vi "Manual Build SM.vi"(8 "error in":errorcluster, 11 "Path to VIPB File":path=path "C:/Users/patrick/Documents/GitHub/PPMS-Monitor-and-Control/build support/PPMS Instrument.vipb") -> (0 "error out":errorcluster)   [LabVIEW 2019]
doc: "JKI State Machine version of Manual Build.vi that also builds a VIPM *.vip file.\n\nUse to build a (0) VI Package, (1) Application (EXE), (2) Installer, and finally (3) a single 7z self-extracting installer file.\n\n<b>Path to VIPB File</b> points to the VI Package Build spec you would like to build. Searchs for *.lvproj."
uses:
  <vilib>/AppBuilder/AB_API_Simple/NI_App_Builder_API.lvlib
  <vilib>/JKI/VIPM API/VIPM API_vipm_api.lvlib
  <userlib>/LevyLab/Progress Bar/ProgressBar/ProgressBar.lvclass
  <vilib>/AppBuilder/AB_API_Simple/Build (path).vi
  <vilib>/AppBuilder/AB_API_Simple/Set Build Specification Version (path).vi
  PostBuildSupport/PostBuildSupport.lvclass
  ProjectItem/ProjectItem.lvclass
  Build/Build.lvlib
panel:
  out "Current State":string="Exit"
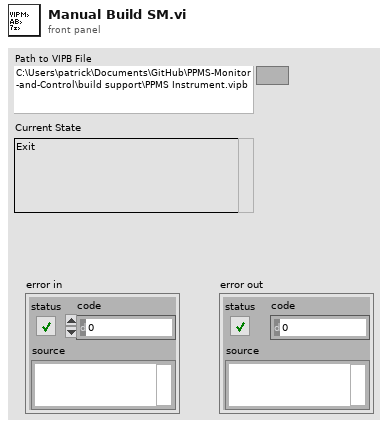
[diagram p1: front panel]
types:
  T1 = enum32{"Invalid", "Standard", "Closed", "Hidden", "Minimized", "Maximized"}
  T2 = enum32{"invalid app kind", "Development System", "Run Time System", "Student Edition", "Embedded LabVIEW", "Evaluation", "Custom"}
  T3 = cluster{"Core":cluster{"Current VI Reference":refnum<vi>, "Close Panel on Exit?":bool}, "ProgressBar":refnum<class "ProgressBar.lvclass">, "Product Name":string, "Package Version":string, "Package Source Folder":path, "Path to Project":path, "Path to VIPB File":path, "Output Package File Path":path}
  T4 = cluster{"Current VI Reference":refnum<vi>, "Close Panel on Exit?":bool}
  T5 = typedef "VIPM API_vipm_api.lvlib/VI Package Build Spec Data Cluster_vipm_api.ctl" = cluster{"Package Version":T6, "Product Name":string, "Company Name":string, "Author Name (Person or Company)":string, "Product Homepage (URL)":string, "Legal Copyright":string, "License Agreement Name":string, "Product Description Summary":string, "Product Description":string, "Release Notes - Change Log":string}
  T6 = typedef "VIPM API_vipm_api.lvlib/Version Info Cluster_vipm_api.ctl" = cluster{"major":u32, "minor":u32, "patch":u32, "build":u32}
  T7 = typedef "Build.lvlib/Build Spec--cluster.ctl" = cluster{"Name":string, "Type":string, "Version":string}
  T8 = typedef "NI_App_Builder_API.lvlib/Build Specification Version.ctl" = cluster{"Major":u16, "Minor":u16, "Fix":u16, "Build":u16}
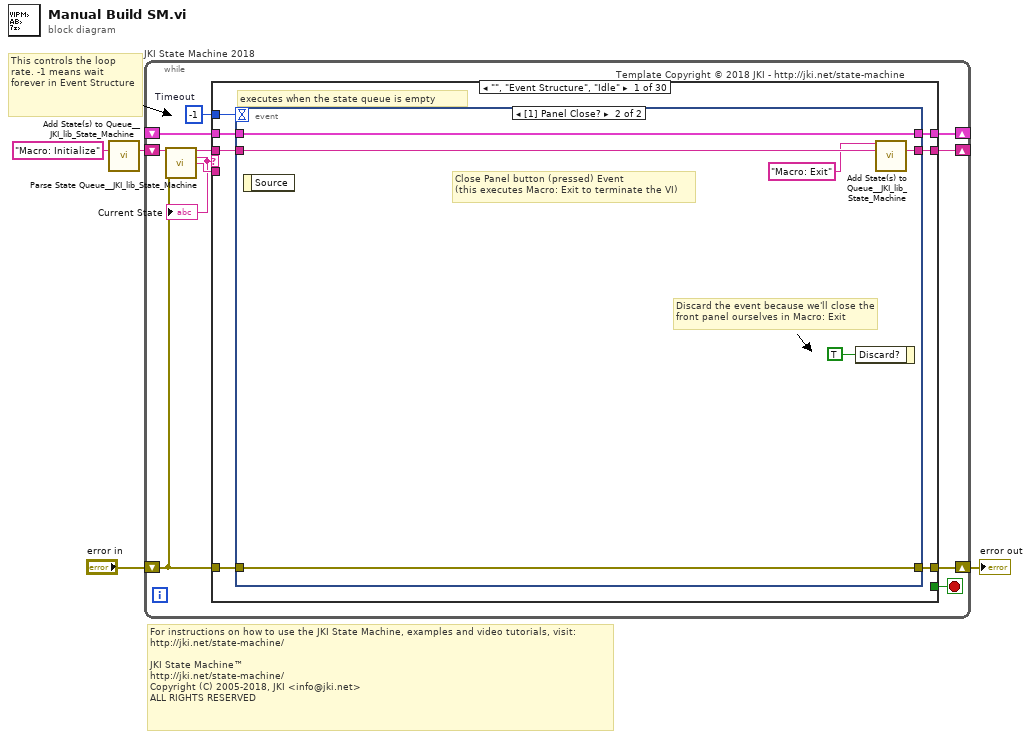
[diagram p0: block diagram]
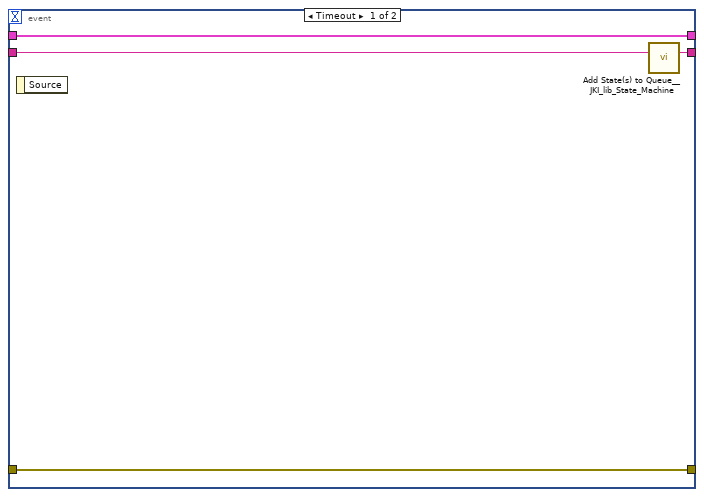
[diagram p2: hidden frame]
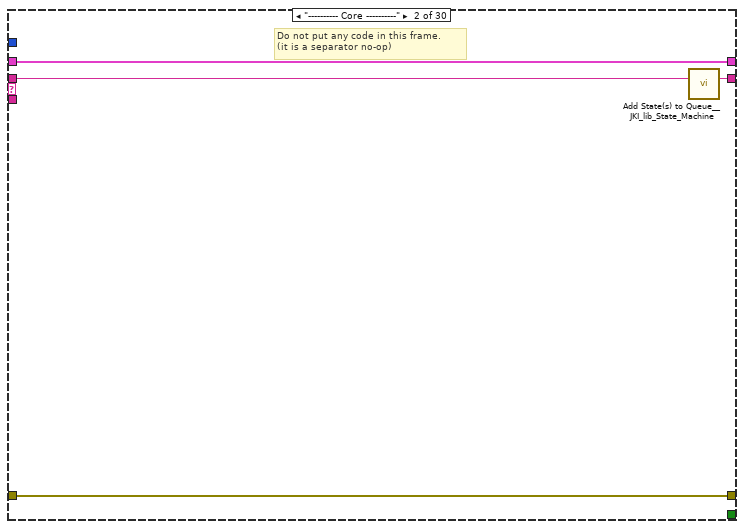
[diagram p3: hidden frame]
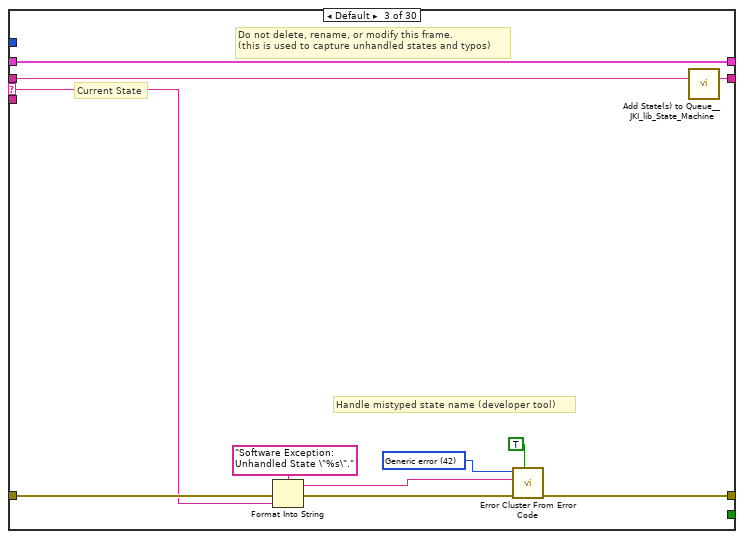
[diagram p4: hidden frame]
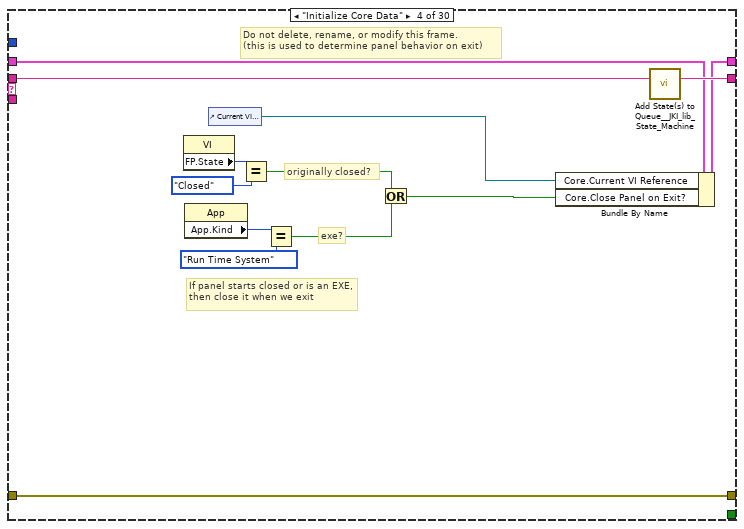
[diagram p5: hidden frame]
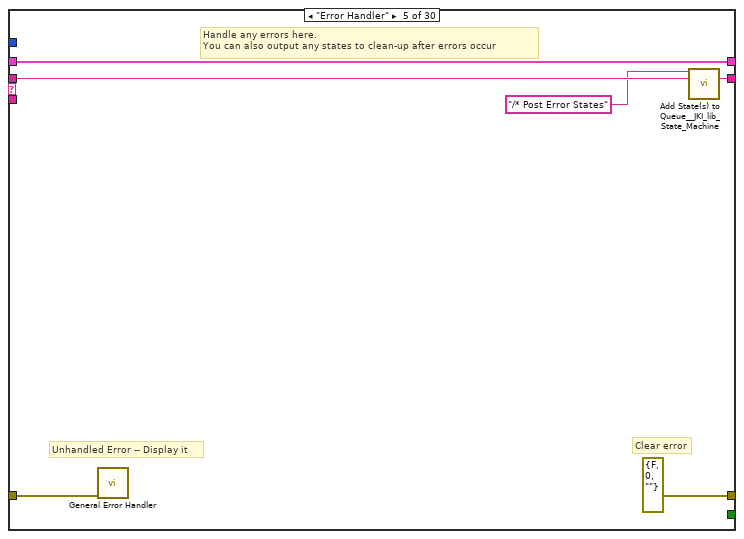
[diagram p6: hidden frame]
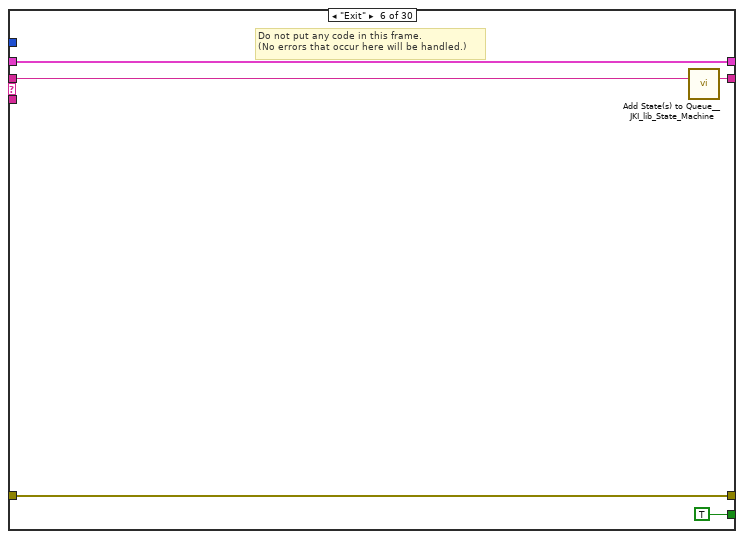
[diagram p7: hidden frame]
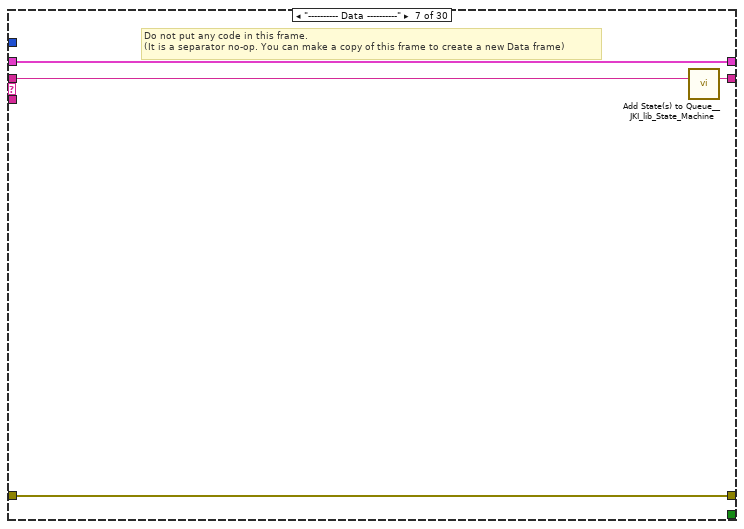
[diagram p8: hidden frame]
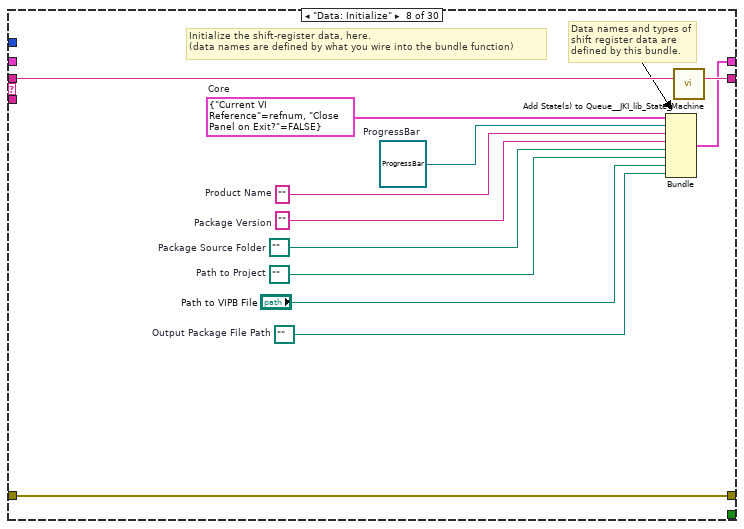
[diagram p9: hidden frame]
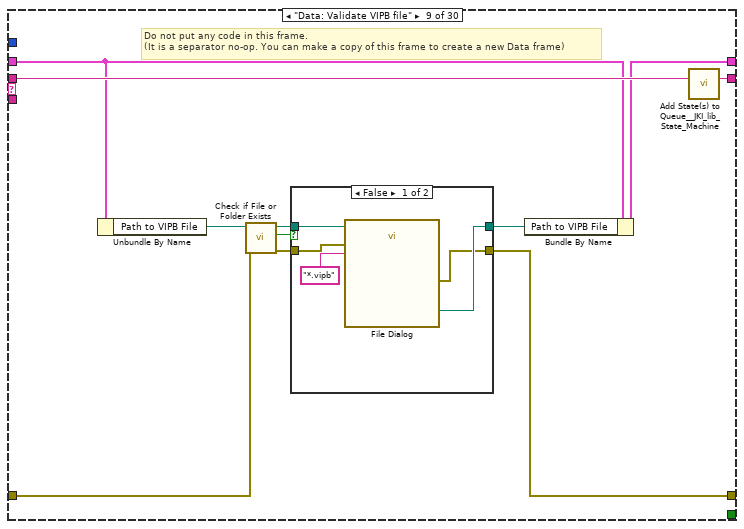
[diagram p10: hidden frame]
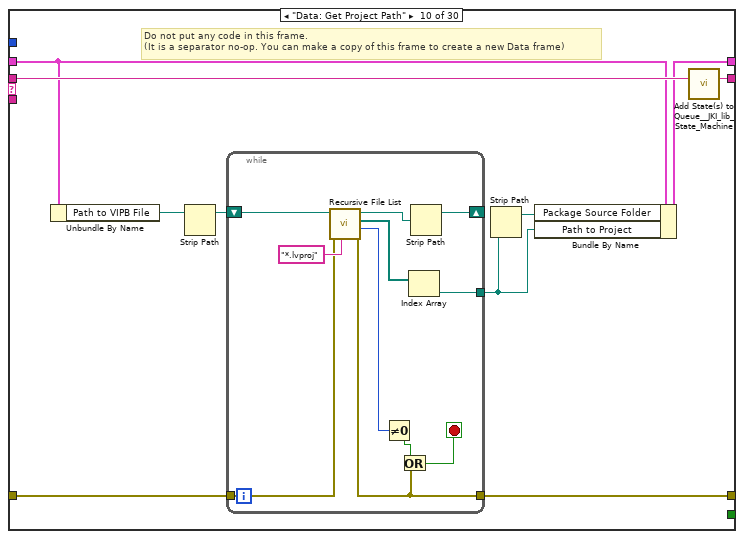
[diagram p12: hidden frame]
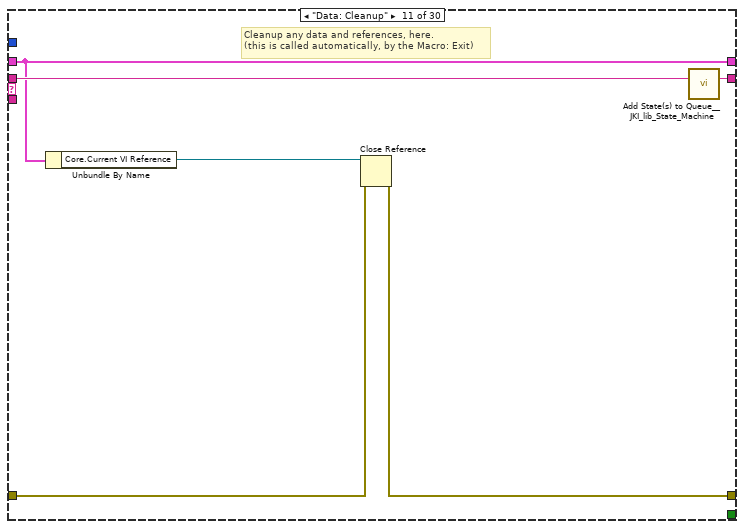
[diagram p13: hidden frame]
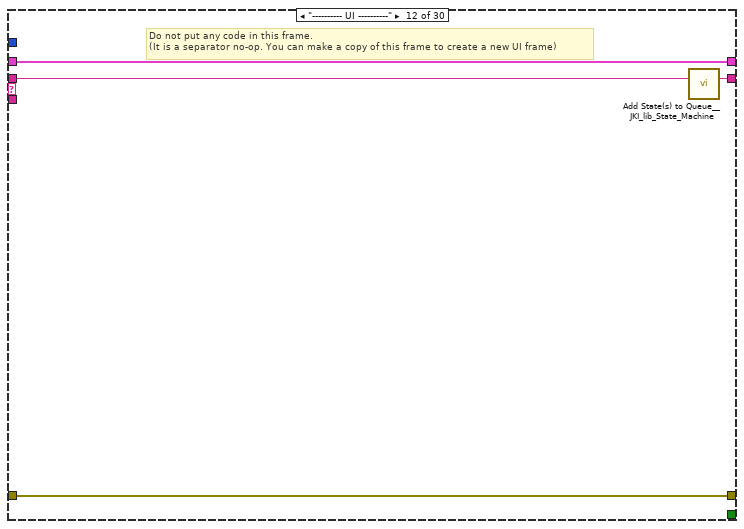
[diagram p14: hidden frame]
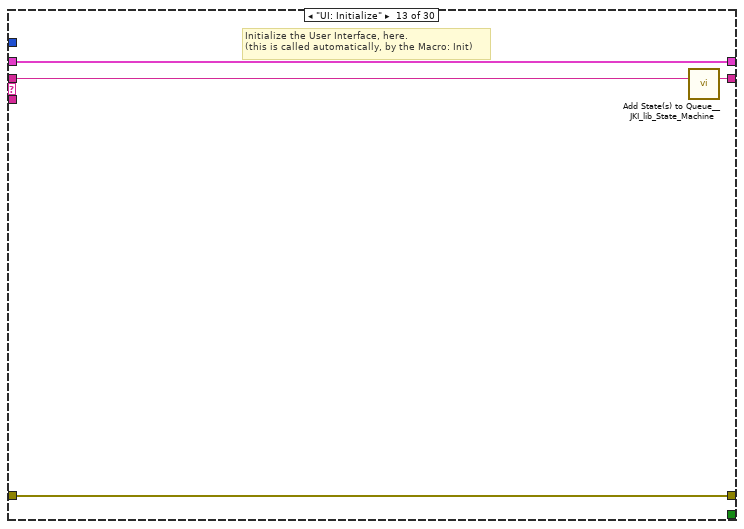
[diagram p15: hidden frame]
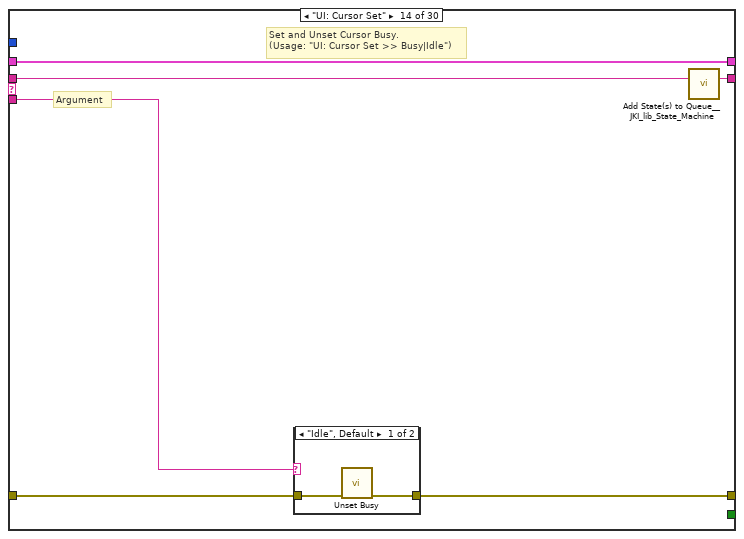
[diagram p16: hidden frame]
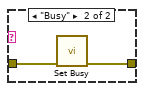
[diagram p17: hidden frame]
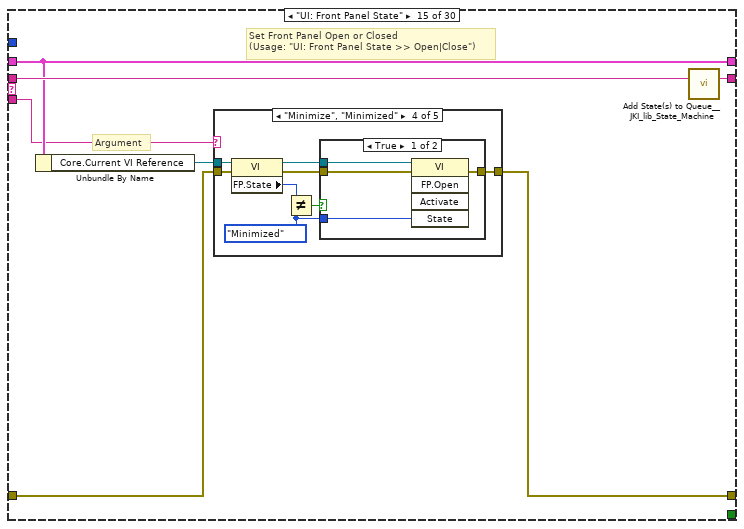
[diagram p18: hidden frame]
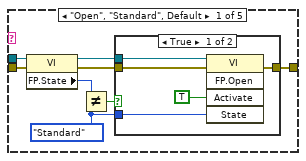
[diagram p19: hidden frame]
diagram:
  # "For instructions on how to use the JKI State Machine, examples and video tutorials, visit:\nhttp://jki.net/state-machine/\n\nJKI State Machine™\nhttp://jki.net/state-machine/\nCopyright (C) 2005-2018, JKI <info@jki.net>\nALL RIGHTS RESERVED"
  # "This controls the loop rate. -1 means wait forever in Event Structure"
  n1 = call <vilib>:"Add State(s) to Queue__JKI_lib_State_Machine.vi"("State(s) in (\"\")"="Macro: Initialize") -> ("States Out"=w4:string)  [unwired: 14 in]
  n2 = while "JKI State Machine 2018" {
    shift-right: [w9] -> _
    shift-left: _ -> [w8]
    shift-right: [w12] -> w2
    shift-left: "error in" -> [w6]
    shift-right: [w11] -> _
    shift-left: w4 -> [w13]
    stop <- w10 stop-if-true
    w7 = -1  # Timeout
    # "Template Copyright © 2018 JKI - http://jki.net/state-machine"
    n3 = call <vilib>:"Parse State Queue__JKI_lib_State_Machine.vi"("State Queue"=w13, "Error In (no error)"=w6) -> ("Remaining States"=w15:string, "Current State"=w5:string, "Arguments"=w14:string)  [unwired: 11 in]
    "Current State" <- w5
    n4 = case shown="\"\", \"Event Structure\", \"Idle\"" w5 {
      selector: w5 -> [_ _ w37 _ _ _ _ _ _ _ _ _ _ _ _ _ _ _ _ _ _ _ _ _ _ _ _ _ w326 _]
      tunnel: w15 -> [w22 w36 w41 w60 w66 w71 w75 w87 w98 w115 w132 w136 w140 w146 w157 w226 w231 w236 w247 w251 w266 w274 w278 w286 w294 w303 w307 w319 w331 w339]
      tunnel: w14 -> [_ _ _ _ _ _ _ _ _ _ _ _ _ w141 w151 _ _ _ _ _ _ _ _ _ _ w295 _ w311 w321 _]
      tunnel: w8 -> [w20 w33 w39 w53 w63 w69 w72 _ w91 w112 w127 w133 w138 w144 w153 w223 w228 w233 w244 w249 w256 w267 w276 w279 w291 w300 w305 w317 w329 w337]
      tunnel: [w19 w34 w43 w57 errorcluster {"status"=FALSE, "code"=0, "source"=""} ("error out") w68 w73 w84 w90 w111 w128 w134 w137 w142 w154 w224 w229 w234 w245 w248 w253 w271 w275 w282 w287 w297 w304 w316 w328 w333] -> w12
      tunnel: w6 -> [w18 w34 w42 w57 w62 w68 w73 w84 w88 w110 w129 w134 w137 w143 w155 w224 w229 w234 w245 w248 w252 w270 w275 w281 w288 w296 w304 w312 w327 _]
      tunnel: [w21 w35 w40 w59 w65 w70 w74 w86 w97 w114 w131 w135 w139 w145 w156 w225 w230 w235 w246 w250 w265 w273 w277 w285 w293 w302 w306 w318 w330 w338] -> w11
      tunnel: [_ _ _ _ _ TRUE _ _ _ _ _ _ _ _ _ _ _ _ _ _ _ _ _ _ _ _ _ _ _ _] -> w10
      tunnel: [w17 w33 w39 w58 w63 w69 w72 w85 w92 w113 w127 w133 w138 w144 w153 w223 w228 w233 w244 w249 w257 w268 w276 w280 w292 w301 w305 w317 w329 w337] -> w9
      tunnel: w7 -> [w16 _ _ _ _ _ _ _ _ _ _ _ _ _ _ _ _ _ _ _ _ _ _ _ _ _ _ _ _ _]
      frame "", "Event Structure", "Idle" {
        # "executes when the state queue is empty"
        n5 = event shown="[1] Panel Close?" {
          selector: _ -> [_ _]
          dyn-events: _ -> [_ _]
          timeout: w16 -> [_ _]
          tunnel: w22 -> [w26 w32]
          tunnel: [w25 w31] -> w21
          tunnel: w20 -> [w23 w29]
          tunnel: [w24 w30] -> w19
          tunnel: w18 -> [w24 w30]
          tunnel: [w23 w29] -> w17
          event Timeout {
            n6 = event-data() -> ()  [unwired: 1 in, 1 out]
            n7 = call <vilib>:"Add State(s) to Queue__JKI_lib_State_Machine.vi"("State(s) in (\"\")"=w26) -> ("States Out"=w25:string)  [unwired: 14 in]
          }
          event Panel Close? {
            # "Discard the event because we'll close the front panel ourselves in Macro: Exit"
            # "Close Panel button (pressed) Event\n(this executes Macro: Exit to terminate the VI)"
            n8 = event-data() -> ()  [unwired: 1 in, 1 out]
            n9 = event-data("Discard?"=TRUE) -> ()  [unwired: 1 in, 1 out]
            n10 = call <vilib>:"Add State(s) to Queue__JKI_lib_State_Machine.vi"("State(s) in Front (\"\")"="Macro: Exit", "State(s) in (\"\")"=w32) -> ("States Out"=w31:string)  [unwired: 13 in]
          }
        }
      }
      frame "---------- Core ----------" {
        # "Do not put any code in this frame.\n(it is a separator no-op)"
        n11 = call <vilib>:"Add State(s) to Queue__JKI_lib_State_Machine.vi"("State(s) in (\"\")"=w36) -> ("States Out"=w35:string)  [unwired: 14 in]
      }
      frame Default {
        w46 = 42 items=["No error", "Argument error", "Memory is full", "Out of zone", "End of file", "File already open", "Generic file I/O error", "File not found", "File permission error", "Disk is full", "Duplicate path", "Too many files open", "System feature not enabled", "Resource file not found", "Cannot add resource", "Resource not found", "Image not found", "Image memory error", "Pen does not exist", "Config type invalid", "Config token not found", "Config parse error", "Config memory error", "Bad external code format", "Bad external code offset", "External code not present", "Null window", "Destroy window error", "Null menu", "Print aborted", "Bad print record", "Print driver error", "Windows error during printing", "Memory error during printing", "Print dialog error", "Generic print error", "Invalid device refnum", "Device not found", "Device parameter error", "Device unit error", "Cannot open device", "Device call aborted", "Generic error", "Cancelled by user", "Object ID too low", "Object ID too high", "Object not in heap", "Unknown heap", "Unknown object (invalid DefProc)", "Unknown object (DefProc not in table)", "Message out of range", "Invalid (null) method", "Unknown message", "Manager call not supported", "Bad address", "Network operation in progress", "Network operation timed out", "Connection is busy", "Network attribute not supported", "Network error", "Address in use", "System out of memory", "Connection aborted", "Connection refused", "Not connected", "Already connected", "Connection closed", "Initialization error (interapplication manager)", "Bad occurrence", "Wait on unbound occurrence handler", "Occurrence queue overflow", "Datalog type conflict", "Unused", "Unrecognized type (interapplication manager)", "Memory corrupt", "Failed to make temporary DLL", "Old CIN version", "Drag socket not found", "Failed to load drop-object", "Failed to register OLE object", "Failed to release OLE object", "Format specifier type mismatch", "Unknown format specifier", "Too few format specifiers", "Too many format specifiers", "Scan failed", "Newer CIN version", "Error converting to variant", "Runtime menu error", "Password tampered", "Variant attribute not found", "Incompatible variant data type", "Event data is not available", "Event Store is not present", "Occurrence is not found", "Event Queue is not created", "Event info is not available", "Refnum passed is NULL", "Error retrieving Class GUID", "Error retrieving CoClass GUID", "Error retrieving TypeLib GUID.", "Bad built application magic bytes.", "Specific driver is different from the specific driver associated with the Logical Name.", "There is no session opened to the class driver.", "Max Error", "MAX - Error with config objects", "MAX - Error loading configuration", "MAX - Group not supported"]
        # "Current State"
        # "Do not delete, rename, or modify this frame.\n(this is used to capture unhandled states and typos)"
        # "Handle mistyped state name (developer tool)"
        n12 = Format Into String(format string="Software Exception: Unhandled State \"%s\"." ("message"), error in=w42, w37) -> (resulting string=w45:string, error out=w44:errorcluster)  [unwired: 1 in]
        n13 = call <vilib>:"Error Cluster From Error Code.vi"("show call chain? (False)"=TRUE, "error in (no error)"=w44, "error message (\"\")"=w45, "error code (0)"=w46) -> ("error out"=w43:errorcluster)  [unwired: 5 in]
        n14 = call <vilib>:"Add State(s) to Queue__JKI_lib_State_Machine.vi"("State(s) in (\"\")"=w41) -> ("States Out"=w40:string)  [unwired: 14 in]
      }
      frame "Initialize Core Data" {
        # "Do not delete, rename, or modify this frame.\n(this is used to determine panel behavior on exit)"
        # "originally closed?"
        # "exe?"
        # "If panel starts closed or is an EXE, then close it when we exit"
        n15 = property class="VI"() -> ("FP.State"=w50:T1)  [unwired: 2 in, 2 out]
        n16 = property class="App"() -> ("App.Kind"=w56:T2)  [unwired: 2 in, 2 out]
        n17 = control-ref of="Current VI Reference"() -> (w51:refnum<vi>)
        n18 = Equal?(x=w50, y=T1."Closed" ("Front Panel Window:State")) -> (x = y?=w48:bool)
        n19 = Equal?(x=w56, y=T2."Run Time System" ("Application:Kind")) -> (x = y?=w54:bool)
        n20 = Or(x=w48, y=w54) -> (x .or. y?=w52:bool)
        n21 = Bundle By Name(cluster=w53, "Core.Current VI Reference"=w51, "Core.Close Panel on Exit?"=w52) -> (w58:T3)
        n22 = call <vilib>:"Add State(s) to Queue__JKI_lib_State_Machine.vi"("State(s) in (\"\")"=w60) -> ("States Out"=w59:string)  [unwired: 14 in]
      }
      frame "Error Handler" {
        # "Unhandled Error -- Display it"
        # "Handle any errors here.\nYou can also output any states to clean-up after errors occur"
        # "Clear error"
        n23 = call <vilib>:"General Error Handler.vi"("error in (no error)"=w62) -> ()  [unwired: 10 in, 5 out]
        n24 = call <vilib>:"Add State(s) to Queue__JKI_lib_State_Machine.vi"("State(s) in Front (\"\")"="/* Post Error States", "State(s) in (\"\")"=w66) -> ("States Out"=w65:string)  [unwired: 13 in]
      }
      frame "Exit" {
        # "Do not put any code in this frame.\n(No errors that occur here will be handled.)"
        n25 = call <vilib>:"Add State(s) to Queue__JKI_lib_State_Machine.vi"("State(s) in (\"\")"=w71) -> ("States Out"=w70:string)  [unwired: 14 in]
      }
      frame "---------- Data ----------" {
        # "Do not put any code in this frame.\n(It is a separator no-op. You can make a copy of this frame to create a new Data frame)"
        n26 = call <vilib>:"Add State(s) to Queue__JKI_lib_State_Machine.vi"("State(s) in (\"\")"=w75) -> ("States Out"=w74:string)  [unwired: 14 in]
      }
      frame "Data: Initialize" {
        w77 = path ""  # Path to Project
        w78 = refnum<class "ProgressBar.lvclass"> refnum  # ProgressBar
        w79 = path ""  # Output Package File Path
        w81 = ""  # Package Version
        w82 = ""  # Product Name
        w80 = path ""  # Package Source Folder
        w83 = T4 {"Current VI Reference"=refnum, "Close Panel on Exit?"=FALSE}  # Core
        # "Data names and types of shift register data are defined by this bundle."
        # "Initialize the shift-register data, here.\n(data names are defined by what you wire into the bundle function)"
        n27 = Bundle("Core"=w83, "ProgressBar"=w78, "Product Name"=w82, "Package Version"=w81, "Package Source Folder"=w80, "Path to Project"=w77, "Path to VIPB File"="Path to VIPB File", "Output Package File Path"=w79) -> (w85:T3)  [unwired: 1 in]
        n28 = call <vilib>:"Add State(s) to Queue__JKI_lib_State_Machine.vi"("State(s) in (\"\")"=w87) -> ("States Out"=w86:string)  [unwired: 14 in]
      }
      frame "Data: Validate VIPB file" {
        # "Do not put any code in this frame.\n(It is a separator no-op. You can make a copy of this frame to create a new Data frame)"
        n29 = Unbundle By Name(w91) -> ("Path to VIPB File"=w95:path)
        n30 = call <vilib>:"Check if File or Folder Exists.vi"("error in (no error)"=w88, "path"=w95) -> ("error out"=w89:errorcluster, "file or folder exists?"=w96:bool, "dup path"=w94:path)  [unwired: 7 in]
        n31 = case shown="False" w96 {
          tunnel: w94 -> [w103 w105]
          tunnel: [w102 w105] -> w93
          tunnel: [w99 w104] -> w90
          tunnel: w89 -> [w101 w104]
          frame False {
            n32 = call "File Dialog"("start path"=w103, "error in"=w101, "pattern (all files)"="*.vipb") -> ("selected path"=w102:path, "error out"=w99:errorcluster)  [unwired: 9 in, 2 out]
          }
          frame True {
          }
        }
        n33 = Bundle By Name(cluster=w91, "Path to VIPB File"=w93) -> (w92:T3)
        n34 = call <vilib>:"Add State(s) to Queue__JKI_lib_State_Machine.vi"("State(s) in (\"\")"=w98) -> ("States Out"=w97:string)  [unwired: 14 in]
      }
      frame "Data: Get Project Path" {
        # "Do not put any code in this frame.\n(It is a separator no-op. You can make a copy of this frame to create a new Data frame)"
        n35 = Unbundle By Name(w112) -> ("Path to VIPB File"=w109:path)
        n36 = Strip Path(path=w109) -> (stripped path=w108:path)  [unwired: 1 out]
        n37 = while {
          tunnel: [w119] -> w111
          tunnel: w110 -> [w121]
          shift-right: [w124] -> _
          shift-left: w108 -> [w120]
          tunnel: [w122] -> w107
          stop <- w117 stop-if-true
          n38 = call <vilib>:"Recursive File List.vi"("pattern"="*.lvproj", "error in (no error)"=w121, "Folder Path"=w120) -> ("error out"=w119:errorcluster, "Number of Files"=w125:i32, "All Files in Dir"=w116:path[], "dup Folder Path"=w123:path)  [unwired: 4 in, 1 out]
          n39 = Not Equal To 0?(x=w125) -> (x != 0?=w118:bool)
          n40 = Or(x=w118, y=w119) -> (x .or. y?=w117:bool)
          n41 = Index Array(array=w116) -> (element=w122:path)  [unwired: 1 in]
          n42 = Strip Path(path=w123) -> (stripped path=w124:path)  [unwired: 1 out]
        }
        n43 = Strip Path(path=w107) -> (stripped path=w106:path)  [unwired: 1 out]
        n44 = Bundle By Name(cluster=w112, "Package Source Folder"=w106, "Path to Project"=w107) -> (w113:T3)
        n45 = call <vilib>:"Add State(s) to Queue__JKI_lib_State_Machine.vi"("State(s) in (\"\")"=w115) -> ("States Out"=w114:string)  [unwired: 14 in]
      }
      frame "Data: Cleanup" {
        # "Cleanup any data and references, here.\n(this is called automatically, by the Macro: Exit)"
        n46 = Unbundle By Name(w127) -> ("Core.Current VI Reference"=w130:refnum<vi>)
        n47 = Close Reference(reference=w130, error in (no error)=w129) -> (error out=w128:errorcluster)
        n48 = call <vilib>:"Add State(s) to Queue__JKI_lib_State_Machine.vi"("State(s) in (\"\")"=w132) -> ("States Out"=w131:string)  [unwired: 14 in]
      }
      frame "---------- UI ----------" {
        # "Do not put any code in this frame.\n(It is a separator no-op. You can make a copy of this frame to create a new UI frame)"
        n49 = call <vilib>:"Add State(s) to Queue__JKI_lib_State_Machine.vi"("State(s) in (\"\")"=w136) -> ("States Out"=w135:string)  [unwired: 14 in]
      }
      frame "UI: Initialize" {
        # "Initialize the User Interface, here.\n(this is called automatically, by the Macro: Init)"
        n50 = call <vilib>:"Add State(s) to Queue__JKI_lib_State_Machine.vi"("State(s) in (\"\")"=w140) -> ("States Out"=w139:string)  [unwired: 14 in]
      }
      frame "UI: Cursor Set" {
        # "Argument"
        # "Set and Unset Cursor Busy.\n(Usage: \"UI: Cursor Set >> Busy|Idle\")"
        n51 = case shown="\"Idle\", Default" w141 {
          tunnel: w143 -> [w148 w150]
          tunnel: [w147 w149] -> w142
          frame "Idle", Default {
            n52 = call <vilib>:"Unset Busy.vi"("error in (no error)"=w148) -> ("error out"=w147:errorcluster)  [unwired: 10 in]
          }
          frame "Busy" {
            n53 = call <vilib>:"Set Busy.vi"("error in (no error)"=w150) -> ("error out"=w149:errorcluster)  [unwired: 9 in, 1 out]
          }
        }
        n54 = call <vilib>:"Add State(s) to Queue__JKI_lib_State_Machine.vi"("State(s) in (\"\")"=w146) -> ("States Out"=w145:string)  [unwired: 14 in]
      }
      frame "UI: Front Panel State" {
        # "Argument"
        # "Set Front Panel Open or Closed\n(Usage: \"UI: Front Panel State >> Open|Close\")"
        n55 = Unbundle By Name(w153) -> ("Core.Current VI Reference"=w152:refnum<vi>)
        n56 = case shown="\"Minimize\", \"Minimized\"" w151 {
          tunnel: w155 -> [w163 w178 w189 w202 w215]
          tunnel: [w165 w179 w191 w204 w217] -> w154
          tunnel: w152 -> [w164 w176 w190 w203 w216]
          frame "Open", "Standard", Default {
            w158 = T1."Standard" ("State")
            n57 = property class="VI"(reference=w164, error in=w163) -> (reference out=w161:refnum<vi>, error out=w162:errorcluster, "FP.State"=w160:T1)
            n58 = Not Equal?(x=w160, y=w158) -> (x != y?=w159:bool)
            n59 = case shown="True" w159 {
              tunnel: [w169 w171] -> w165
              tunnel: w162 -> [w168 w171]
              tunnel: w161 -> [w167 _]
              tunnel: w158 -> [w166 _]
              frame True {
                n60 = invoke class="VI" method="FP.Open"(reference=w167, error in=w168, "Activate"=TRUE, "State"=w166) -> (error out=w169:errorcluster)  [unwired: 1 in, 4 out]
              }
              frame False {
              }
            }
          }
          frame "Close", "Closed" {
            n61 = property class="VI"(reference=w176, error in=w178) -> (reference out=w175:refnum<vi>, error out=w177:errorcluster, "FP.State"=w173:T1)
            n62 = Not Equal?(x=w173, y=T1."Closed" ("Front Panel Window:State")) -> (x != y?=w172:bool)
            n63 = case shown="True" w172 {
              tunnel: [w180 w183] -> w179
              tunnel: w177 -> [w180 w182]
              tunnel: w175 -> [_ w181]
              frame False {
              }
              frame True {
                n64 = invoke class="VI" method="FP.Close"(reference=w181, error in=w182) -> (error out=w183:errorcluster)  [unwired: 1 in, 2 out]
              }
            }
          }
          frame "Hidden", "Hide" {
            w184 = T1."Hidden" ("State")
            n65 = property class="VI"(reference=w190, error in=w189) -> (reference out=w187:refnum<vi>, error out=w188:errorcluster, "FP.State"=w186:T1)
            n66 = Not Equal?(x=w186, y=w184) -> (x != y?=w185:bool)
            n67 = case shown="True" w185 {
              tunnel: [w195 w196] -> w191
              tunnel: w188 -> [w194 w196]
              tunnel: w187 -> [w193 _]
              tunnel: w184 -> [w192 _]
              frame True {
                n68 = invoke class="VI" method="FP.Open"(reference=w193, error in=w194, "State"=w192) -> (error out=w195:errorcluster)  [unwired: 2 in, 4 out]
              }
              frame False {
              }
            }
          }
          frame "Minimize", "Minimized" {
            w197 = T1."Minimized" ("State")
            n69 = property class="VI"(reference=w203, error in=w202) -> (reference out=w200:refnum<vi>, error out=w201:errorcluster, "FP.State"=w199:T1)
            n70 = Not Equal?(x=w199, y=w197) -> (x != y?=w198:bool)
            n71 = case shown="True" w198 {
              tunnel: [w208 w209] -> w204
              tunnel: w201 -> [w207 w209]
              tunnel: w200 -> [w206 _]
              tunnel: w197 -> [w205 _]
              frame True {
                n72 = invoke class="VI" method="FP.Open"(reference=w206, error in=w207, "State"=w205) -> (error out=w208:errorcluster)  [unwired: 2 in, 4 out]
              }
              frame False {
              }
            }
          }
          frame "Maximize", "Maximized" {
            w210 = T1."Maximized" ("State")
            n73 = property class="VI"(reference=w216, error in=w215) -> (reference out=w213:refnum<vi>, error out=w214:errorcluster, "FP.State"=w212:T1)
            n74 = Not Equal?(x=w212, y=w210) -> (x != y?=w211:bool)
            n75 = case shown="True" w211 {
              tunnel: [w221 w222] -> w217
              tunnel: w214 -> [w220 w222]
              tunnel: w213 -> [w219 _]
              tunnel: w210 -> [w218 _]
              frame True {
                n76 = invoke class="VI" method="FP.Open"(reference=w219, error in=w220, "State"=w218) -> (error out=w221:errorcluster)  [unwired: 2 in, 4 out]
              }
              frame False {
              }
            }
          }
        }
        n77 = call <vilib>:"Add State(s) to Queue__JKI_lib_State_Machine.vi"("State(s) in (\"\")"=w157) -> ("States Out"=w156:string)  [unwired: 14 in]
      }
      frame "---------- Macro ----------" {
        # "Do not put any code in this frame.\n(It is a separator no-op. You can make a copy of this frame to create a new Macro frame)"
        n78 = call <vilib>:"Add State(s) to Queue__JKI_lib_State_Machine.vi"("State(s) in (\"\")"=w226) -> ("States Out"=w225:string)  [unwired: 14 in]
      }
      frame "Macro: Initialize" {
        w227 = "Data: Initialize\nInitialize Core Data\nUI: Initialize\nUI: Front Panel State >> Open\nData: Validate VIPB file\n\nMacro: Build\nMacro: Exit"  # Data: Initialize Initialize Core Data UI: Initialize UI: Front Panel State >> Open Data: Validate VIPB file  Macro: Build Macro: Exit
        # "Initialization Macro\n(This is called once, when the VI starts)"
        n79 = call <vilib>:"Add State(s) to Queue__JKI_lib_State_Machine.vi"("State(s) in Front (\"\")"=w227, "State(s) in (\"\")"=w231) -> ("States Out"=w230:string)  [unwired: 13 in]
      }
      frame "Macro: Build" {
        # "Initialization Macro\n(This is called once, when the VI starts)"
        n80 = call <vilib>:"Add State(s) to Queue__JKI_lib_State_Machine.vi"("State(s) in Front (\"\")"="Data: Get Project Path\nVIPM: Read VIPB\nVIPM: Build\nAB: Update Version >> Application\nAB: Update Version >> Installer\nAB: Build >> Application\nAB: Build >> Installer\nAB: Build exe", "State(s) in (\"\")"=w236) -> ("States Out"=w235:string)  [unwired: 13 in]
      }
      frame "Macro: Exit" {
        # "Exit Macro\n(This is called once, when the VI exits)"
        n81 = Unbundle By Name(w244) -> ("Core.Close Panel on Exit?"=w243:bool)
        n82 = Select(t="UI: Front Panel State >> Close", s=w243, f="") -> (s? t:f=w240:string)
        n83 = call <vilib>:"Add State(s) to Queue__JKI_lib_State_Machine.vi"("State(s) in Front (\"\")"="", "State(s) in (\"\")"=w240, "State(s) at Back (\"\")"="Data: Cleanup\nExit") -> ("States Out"=w238:string)  [unwired: 12 in]
        n84 = call <vilib>:"Add State(s) to Queue__JKI_lib_State_Machine.vi"("State(s) in Front (\"\")"=w238, "State(s) in (\"\")"=w247) -> ("States Out"=w246:string)  [unwired: 13 in]
      }
      frame "---------- VIPM ----------" {
        # "Template Separator\n(You can make a copy of, or modify, this frame)"
        n85 = call <vilib>:"Add State(s) to Queue__JKI_lib_State_Machine.vi"("State(s) in (\"\")"=w251) -> ("States Out"=w250:string)  [unwired: 14 in]
      }
      frame "VIPM: Read VIPB" {
        # "Your code here.\n(You can make a copy of, or modify, this frame)"
        n86 = Unbundle By Name(w256) -> ("Path to VIPB File"=w259:path)
        n87 = call <vilib>:"Read VI Package Build Spec_vipm_api.vi"("error in (no error)"=w252, "Path to VIPB File"=w259) -> ("error out"=w253:errorcluster, "VI Package Build Spec Data"=w264:T5)  [unwired: 8 in]
        n88 = Unbundle By Name(w264) -> ("Package Version.major"=w255:u32, "Package Version.minor"=w263:u32, "Package Version.patch"=w262:u32, "Package Version.build"=w261:u32, "Product Name"=w254:string)
        n89 = Format Into String(format string="%d.%d.%d.%d", w255, w263, w262, w261) -> (resulting string=w258:string)  [unwired: 2 in, 1 out]
        n90 = Bundle By Name(cluster=w256, "Package Version"=w258, "Product Name"=w254) -> (w257:T3)
        n91 = call <vilib>:"Add State(s) to Queue__JKI_lib_State_Machine.vi"("State(s) in (\"\")"=w266) -> ("States Out"=w265:string)  [unwired: 14 in]
      }
      frame "VIPM: Build" {
        # "Your code here.\n(You can make a copy of, or modify, this frame)"
        n92 = Unbundle By Name(w267) -> ("Path to VIPB File"=w272:path)
        n93 = call <vilib>:"Build VI Package_vipm_api.vi"("error in (no error)"=w270, "Path to VIPB File"=w272) -> ("error out"=w271:errorcluster, "Build Output"=w269:path)  [unwired: 8 in]
        n94 = Bundle By Name(cluster=w267, "Output Package File Path"=w269) -> (w268:T3)
        n95 = call <vilib>:"Add State(s) to Queue__JKI_lib_State_Machine.vi"("State(s) in (\"\")"=w274) -> ("States Out"=w273:string)  [unwired: 14 in]
      }
      frame "---------- ProgressBar ----------" {
        # "Template Separator\n(You can make a copy of, or modify, this frame)"
        n96 = call <vilib>:"Add State(s) to Queue__JKI_lib_State_Machine.vi"("State(s) in (\"\")"=w278) -> ("States Out"=w277:string)  [unwired: 14 in]
      }
      frame "ProgressBar: Initialize" {
        # "Do not put any code in this frame.\n(It is a separator no-op. You can make a copy of this frame to create a new Data frame)"
        n97 = Unbundle By Name(w279) -> ("ProgressBar"=w284:refnum<class "ProgressBar.lvclass">)
        n98 = call <userlib>:"Initialize ProgressBar.vi"("error in (no error)"=w281, "ProgressBar in"=w284) -> ("error out"=w282:errorcluster, "ProgressBar out"=w283:refnum<class "ProgressBar.lvclass">)  [unwired: 8 in]
        n99 = Bundle By Name(cluster=w279, "ProgressBar"=w283) -> (w280:T3)
        n100 = call <vilib>:"Add State(s) to Queue__JKI_lib_State_Machine.vi"("State(s) in (\"\")"=w286) -> ("States Out"=w285:string)  [unwired: 14 in]
      }
      frame "ProgressBar: Destroy" {
        # "Do not put any code in this frame.\n(It is a separator no-op. You can make a copy of this frame to create a new Data frame)"
        n101 = Unbundle By Name(w291) -> ("ProgressBar"=w290:refnum<class "ProgressBar.lvclass">)
        n102 = call <userlib>:"Destroy ProgressBar.vi"("error in (no error)"=w288, "ProgressBar in"=w290) -> ("error out"=w287:errorcluster, "ProgressBar out"=w289:refnum<class "ProgressBar.lvclass">)  [unwired: 8 in]
        n103 = Bundle By Name(cluster=w291, "ProgressBar"=w289) -> (w292:T3)
        n104 = call <vilib>:"Add State(s) to Queue__JKI_lib_State_Machine.vi"("State(s) in (\"\")"=w294) -> ("States Out"=w293:string)  [unwired: 14 in]
      }
      frame "ProgressBar: Update" {
        # "Template Separator\n(You can make a copy of, or modify, this frame)"
        n105 = Unbundle By Name(w300) -> ("ProgressBar"=w299:refnum<class "ProgressBar.lvclass">)
        n106 = call <userlib>:"Send Progress and Message.vi"("error in (no error)"=w296, "Message"=w295, "ProgressBar in"=w299) -> ("error out"=w297:errorcluster, "ProgressBar out"=w298:refnum<class "ProgressBar.lvclass">)  [unwired: 7 in]
        n107 = Bundle By Name(cluster=w300, "ProgressBar"=w298) -> (w301:T3)
        n108 = call <vilib>:"Add State(s) to Queue__JKI_lib_State_Machine.vi"("State(s) in (\"\")"=w303) -> ("States Out"=w302:string)  [unwired: 14 in]
      }
      frame "---------- AB ----------" {
        # "Template Separator\n(You can make a copy of, or modify, this frame)"
        n109 = call <vilib>:"Add State(s) to Queue__JKI_lib_State_Machine.vi"("State(s) in (\"\")"=w307) -> ("States Out"=w306:string)  [unwired: 14 in]
      }
      frame "AB: Update Version" {
        # "Template Separator\n(You can make a copy of, or modify, this frame)"
        n110 = Unbundle By Name(w317) -> ("Path to Project"=w314:path, "Package Version"=w309:string)  [unwired: 1 out]
        n111 = call "List Project Build Specifications.vi"("error in (no error)"=w312, "project path"=w314) -> ("error out"=w313:errorcluster, "Build Specs"=w315:T7[])  [unwired: 8 in]
        n112 = call "Choose Build Spec.vi"("Build Type"=w311, "Build Specs"=w315) -> ("Name"=w310:string)  [unwired: 6 in, 3 out]
        n113 = call "Version String to Build Spec Version.vi"("Package Version"=w309) -> ("Build Specification Version"=w308:T8)
        n114 = call-poly <vilib>:"Set Build Specification Version.vi"("Build Specification Version"=w308, "error in (no error)"=w313, "Name of build specification"=w310, "Path to project"=w314) -> ("error out"=w316:errorcluster)  [unwired: 7 in]
        n115 = call <vilib>:"Add State(s) to Queue__JKI_lib_State_Machine.vi"("State(s) in (\"\")"=w319) -> ("States Out"=w318:string)  [unwired: 14 in]
      }
      frame "AB: Build" {
        # "Template Separator\n(You can make a copy of, or modify, this frame)"
        n116 = Unbundle By Name(w329) -> ("Path to Project"=w322:path)
        n117 = Format Into String(format string="%s %s", w326, w321) -> (resulting string=w325:string)  [unwired: 2 in, 1 out]
        n118 = call "List Project Build Specifications.vi"("project path"=w322) -> ("Build Specs"=w323:T7[])  [unwired: 9 in, 1 out]
        n119 = local write "Current State"(w325) -> ()
        n120 = call "Choose Build Spec.vi"("Build Type"=w321, "Build Specs"=w323) -> ("Name"=w320:string)  [unwired: 6 in, 3 out]
        n121 = call-poly <vilib>:"Build.vi"("error in (no error)"=w327, "Name of build specification (if empty: build all)"=w320, "Path to project"=w322) -> ("error out"=w328:errorcluster)  [unwired: 7 in, 1 out]
        n122 = call <vilib>:"Add State(s) to Queue__JKI_lib_State_Machine.vi"("State(s) in (\"\")"=w331) -> ("States Out"=w330:string)  [unwired: 14 in]
      }
      frame "AB: Build exe" {
        # "build 7z self-extracting installer"
        # "Template Separator\n(You can make a copy of, or modify, this frame)"
        n123 = Unbundle By Name(w337) -> ("Output Package File Path"=w336:path, "Product Name"=w334:string, "Package Version"=w332:string, "Package Source Folder"=w335:path)
        n124 = call "Post Build Script (manual build).vi"("Package Source Folder"=w335, "Package Version"=w332, "Product Name"=w334, "Output Package File Path"=w336) -> ("error out"=w333:errorcluster)  [unwired: 7 in]
        n125 = call <vilib>:"Add State(s) to Queue__JKI_lib_State_Machine.vi"("State(s) in (\"\")"=w339) -> ("States Out"=w338:string)  [unwired: 14 in]
      }
    }
  }
  "error out" <- w2
